vi "ZE_Recorder_Initalize.vi"(8 "error in (no error)":errorcluster, 9 "Button References":refnum<vi>[](array[refnum]), 10 "VI reference in":refnum<vi>, 11 "This Application":refnum<vi>) -> (0 "error out":errorcluster={"status"=TRUE, "code"=1, "source"="Close Reference in ZE_Recorder_Initalize.vi"}, 2 "Action":T7=enum."Error", 3 "output cluster":T1={"Button References"=[], "is recording?"=FALSE, "Header Cluster"={"Project"="", "Operator ID"="", "Description"="Measurement Description: "}, "Channel Array"=[], "File Cluster"={"File Name"="", "File Path Base"=path "", "File Type"=enum."CSV", "Timestamp"=""}, "No of channels"=0, "CSV refnum"=refnum, "tdms refnum"=refnum, "No of samples written"=0, "TDMS channel array"=[], "max Range"=0.0, "sampling rate"=100.0, "ACK Tasks"=[], "multi Device"=FALSE} {"Channel Array"."Terminal" items=["Default"=-1, "RSE"=10083, "NRSE"=10078, "Differential"=10106, "Pseudodifferential"=12529]; "Channel Array"."Range (+/-)" min=-10.0 max=10.0 step=0.1 format="%#_13g"})   [LabVIEW 2019]
doc: "ZE_Recorder_Initalize.vi\n----------------------------------------------\nThis VI initalizes the Recorder and sets controls to default values. The VI also reads the last known set of parameters and applies those to the controls.\n\nInputs:\n---------------------\n- error in (no error) : Cluster; \n- Button References : 1DArrayOfRefnum; \n- VI reference in : Refnum; \n- This Application : Refnum; \n\nOutputs:\n---------------------\n- error out : Cluster; \n- Action : EnumU16; \n- output cluster : Cluster; \n\n----------------------------------------------\n02.06.2016\nZühlke Engineering AG\nCH-8952 Schlieren\nwww.zuehlke.com"
uses:
  TypeDefs/ZE_Recorder_States.ctl
  Libraries/ZE_Recorder/ZE_Recorder.lvlib
  TypeDefs/ZE_Recorder_Header.ctl
  TypeDefs/ZE_Recorder_Units.ctl
  TypeDefs/ZE_Recorder_ChannelCluster.ctl
  TypeDefs/ZE_Recorder_FileCluster.ctl
  TypeDefs/ZE_Recorder_DataCluster.ctl
  TypeDefs/Temperature.ctl
panel:
  in  "?":T1={"Button References"=[], "is recording?"=FALSE, "Header Cluster"={"Project"="", "Operator ID"="", "Description"="Measurement Description: "}, "Channel Array"=[], "File Cluster"={"File Name"="", "File Path Base"=path "", "File Type"=enum."CSV", "Timestamp"=""}, "No of channels"=0, "CSV refnum"=refnum, "tdms refnum"=refnum, "No of samples written"=0, "TDMS channel array"=[], "max Range"=0.0, "sampling rate"=0.0, "ACK Tasks"=[], "multi Device"=FALSE} {"Channel Array"."Terminal" items=["Default"=-1, "RSE"=10083, "NRSE"=10078, "Differential"=10106, "Pseudodifferential"=12529]; "Channel Array"."Range (+/-)" min=-10.0 max=10.0 step=0.1 format="%#_13g"}
  # "Connector Pane"
  # "Locals"
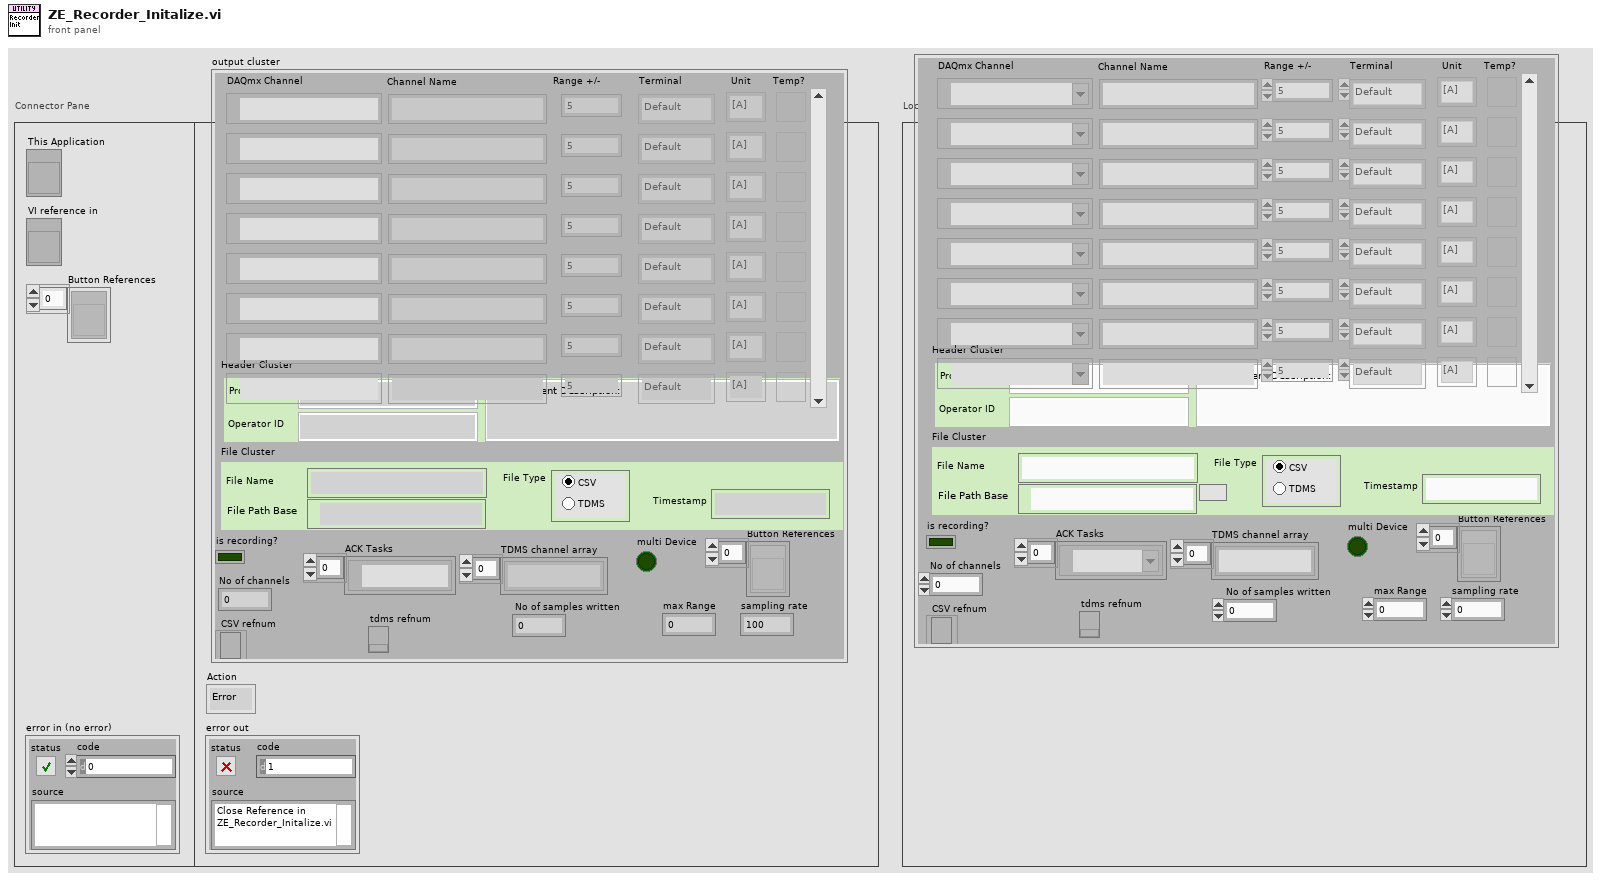
[diagram p1: front panel]
types:
  T1 = typedef "ZE_Recorder.lvlib/ZE_Recorder_DataCluster.ctl" = cluster{"Button References":refnum<vi>[], "is recording?":bool, "Header Cluster":T2, "Channel Array":T3, "File Cluster":T6, "No of channels":i16, "CSV refnum":refnum<file>, "tdms refnum":refnum<k34>, "No of samples written":i64, "TDMS channel array":string[], "max Range":dbl, "sampling rate":dbl, "ACK Tasks":refnum<k21>[], "multi Device":bool}
  T2 = typedef "ZE_Recorder.lvlib/ZE_Recorder_Header.ctl" = cluster{"Project":string, "Operator ID":string, "Description":string}
  T3 = typedef "ZE_Recorder.lvlib/ZE_Recorder_ChannelCluster.ctl" = cluster{"channel name":string, "Unit":T4, "physical channel":tag, "Range (+/-)":dbl, "Terminal":i32, "isTemp":T5}[]
  T4 = typedef "ZE_Recorder.lvlib/ZE_Recorder_Units.ctl" = enum16{"[V]", "[A]", "[F]", "[H]", "[°C]", "[ml/s]", "[m/s]", "[bar]", "[%]", "[N]", "[?]"}
  T5 = typedef "ZE_Recorder.lvlib/Temperature.ctl" = bool
  T6 = typedef "ZE_Recorder.lvlib/ZE_Recorder_FileCluster.ctl" = cluster{"File Name":string, "File Path Base":path, "File Type":enum32{"CSV", "TDMS"}, "Timestamp":string}
  T7 = typedef "ZE_Recorder_States.ctl" = enum16{"Idle", "Error", "Exit VI", "------------<Task>-------------", "Create Tasks", "Release Tasks", "----------<Record>------------", "Close File", "Create File", "Read and Write Data", "Stop Recording", "Start Recording"}
  T8 = enum8{"Enabled", "Disabled", "Disabled and Grayed Out"}
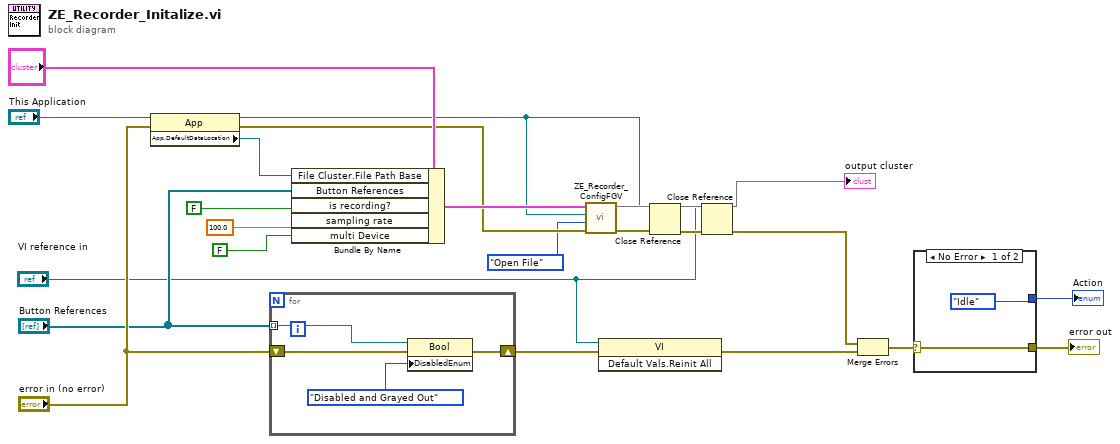
[diagram p0: block diagram]
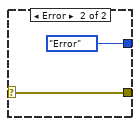
[diagram p2: hidden frame]
diagram:
  n1 = property class="App"(reference="This Application", error in="error in (no error)") -> (reference out=w5:refnum<vi>, error out=w11:errorcluster, "App.DefaultDataLocation"=w19:path)
  n2 = for {
    tunnel: "Button References" -> [w26] mode=indexing
    shift-right: [w24] -> w20
    shift-left: "error in (no error)" -> [w25]
    n3 = property class="Bool"(reference=w26, error in=w25, "DisabledEnum"=T8."Disabled and Grayed Out" ("Disabled")) -> (error out=w24:errorcluster)  [unwired: 1 out]
  }
  n4 = Bundle By Name(cluster="?", "File Cluster.File Path Base"=w19, "Button References"="Button References", "is recording?"=FALSE, "sampling rate"=100.0, "multi Device"=FALSE) -> (w12:T1)
  n5 = call "ZE_Recorder_ConfigFGV.vi"("error in"=w11, "Action"=enum16{"Write and Close File", "Open File"}."Open File", "Application in"=w5, 11:w12) -> ("error out"=w8:errorcluster, 3:→"output cluster")  [unwired: 5 in, 1 out]
  n6 = invoke class="VI" method="Default Vals.Reinit All"(reference="VI reference in", error in=w20) -> (error out=w1:errorcluster)  [unwired: 1 in, 2 out]
  n7 = Close Reference(reference=w5, error in (no error)=w8) -> (error out=w7:errorcluster)
  n8 = Close Reference(reference="VI reference in", error in (no error)=w7) -> (error out=w6:errorcluster)
  n9 = Merge Errors(w6, w1) -> (w16:errorcluster)
  n10 = case shown="No Error" w16 {
    selector: w16 -> [w28 w30]
    tunnel: [w28 w30] -> w15
    tunnel: [ZE_Recorder_States."Idle" ("Action") ZE_Recorder_States."Error" ("Action")] -> w14
    frame No Error {
    }
    frame Error {
    }
  }
  "error out" <- w15
  "Action" <- w14
